vi "WPI_SolenoidSafetyConfig.vi"(8 "error in (no error)":errorcluster, 9 "timeout (s)":dbl=0.1, 10 "mode":T1, 11 "SolenoidDevRef":T2={"DevStatus"={"status"=FALSE, "code"=0, "source"=""}, "Pneumatics Control Module"=0, "Forward Solenoid Channel"=enum."Solenoid 1", "Reverse Solenoid Channel"=enum."Invalid"}) -> (0 "error out":errorcluster, 3 "SolenoidDevRef":T2={"DevStatus"={"status"=FALSE, "code"=0, "source"=""}, "Pneumatics Control Module"=0, "Forward Solenoid Channel"=enum."Solenoid 1", "Reverse Solenoid Channel"=enum."Invalid"})   [LabVIEW 2017]
doc: "Resets the solenoid to its default value if the solenoid does not receive updates faster than the <b>timeout (s)</b> value. This VI is a safety feature to ensure the robot responds to input values, such as joystick values.\n\nThis software is licensed. Open the labview\\readme\\WPI Robotics Library Open Source License.txt file for more information."
uses:
  <vilib>/Rock Robotics/WPI/Solenoid/WPI_SolenoidDevRef.ctl
  <vilib>/Rock Robotics/WPI/Solenoid/WPI_SolenoidChannel.ctl
  <vilib>/Rock Robotics/WPI/SafetyOutput/WPI_SafetyOutputConfigMenu.ctl
  <vilib>/Rock Robotics/WPI/SafetyOutput/WPI_SafetyOutputCheckMenu.ctl
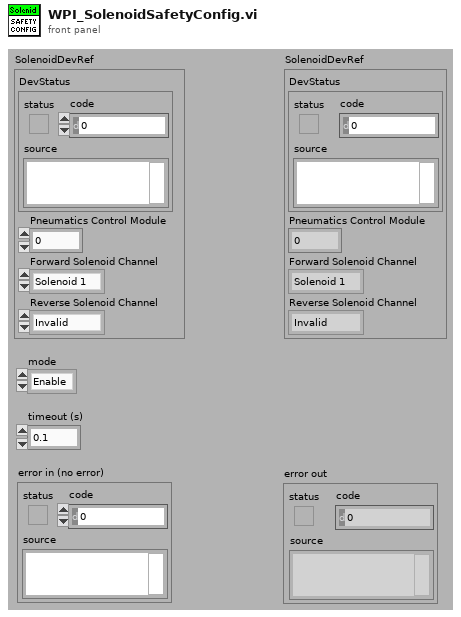
[diagram p1: front panel]
types:
  T1 = typedef "WPI_SafetyOutputConfigMenu.ctl" = enum16{"Enable", "Disable"}
  T2 = typedef "WPI_SolenoidDevRef.ctl" = cluster{"DevStatus":errorcluster, "Pneumatics Control Module":u8, "Forward Solenoid Channel":T3, "Reverse Solenoid Channel":T3}
  T3 = typedef "WPI_SolenoidChannel.ctl" = enum8{"Solenoid 0", "Solenoid 1", "Solenoid 2", "Solenoid 3", "Solenoid 4", "Solenoid 5", "Solenoid 6", "Solenoid 7", "Invalid"}
  T4 = typedef "WPI_SafetyOutputCheckMenu.ctl" = enum16{"test", "add", "remove", "update"}
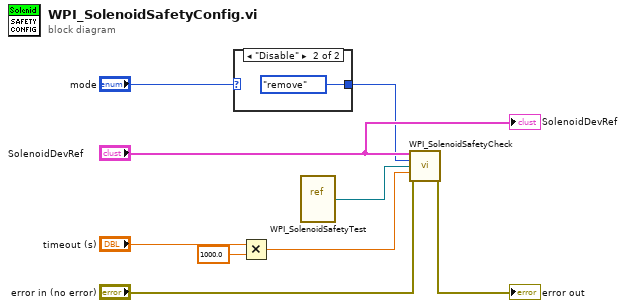
[diagram p0: block diagram]
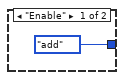
[diagram p2: hidden frame]
diagram:
  n1 = case shown="\"Disable\"" "mode" {
    tunnel: [WPI_SafetyOutputCheckMenu."add" ("menu") WPI_SafetyOutputCheckMenu."remove" ("menu")] -> w4
    frame "Enable" {
    }
    frame "Disable" {
    }
  }
  n2 = Multiply(x="timeout (s)", y=1000.0) -> (x*y=w2:dbl)
  n3 = vi-ref <vilib>:"WPI_SolenoidSafetyTest.vi"() -> (w3:refnum<vi>)
  n4 = call <vilib>:"WPI_SolenoidSafetyCheck.vi"("SolenoidDevRef"="SolenoidDevRef", "menu"=w4, "VI Refnum"=w3, "timeout (ms)"=w2, "error in (no error)"="error in (no error)") -> ("error out"=→"error out":errorcluster)  [unwired: 10 out]
  "SolenoidDevRef" <- "SolenoidDevRef"
